vi "read_new_data.vi"(8 "Error In":errorcluster, 9 "connected?":bool, 10 "VISA in":refnum<visa-resource-name>, 11 "Data Cluster In":T1) -> (0 "error out":errorcluster, 2 "VISA out":refnum<visa-resource-name>, 3 "Data Cluster Out":T1)   [LabVIEW 2021]
uses:
  data_cluster_typedef.ctl
panel:
  out "Serial Settings:Number of Bytes at Serial Port":u32
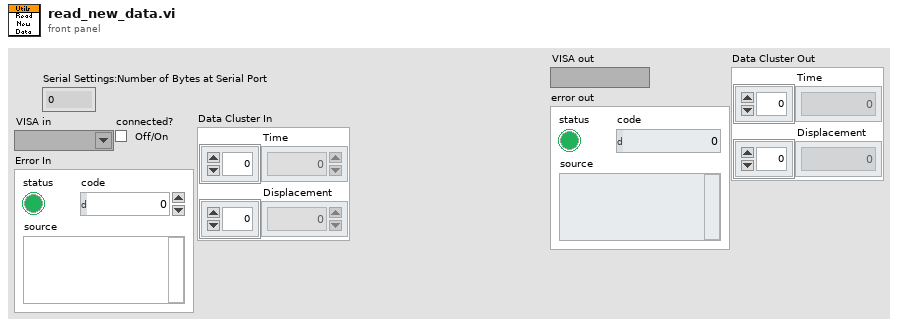
[diagram p1: front panel]
types:
  T1 = typedef "data_cluster_typedef.ctl" = cluster{"Time":dbl[], "Displacement":dbl[]}
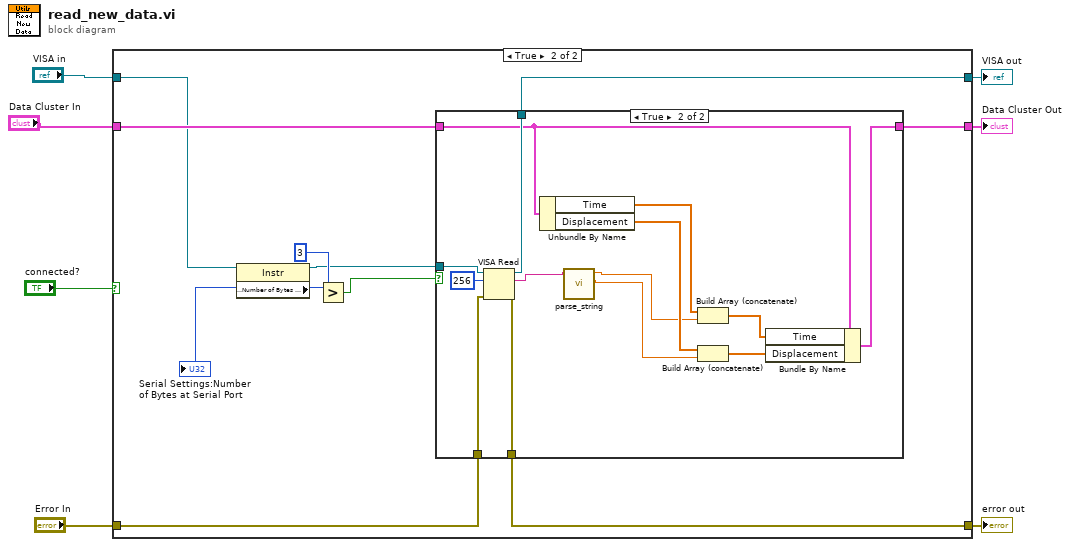
[diagram p0: block diagram]
diagram:
  n1 = case shown="True" "connected?" {
    tunnel: [w10 w20] -> w7
    tunnel: "VISA in" -> [w10 w15]
    tunnel: "Data Cluster In" -> [w9 w18]
    tunnel: [w9 w17] -> w3
    tunnel: "Error In" -> [w8 w19]
    tunnel: [w8 w16] -> w4
    frame False {
      # "Not connected - so just keep passing everything\nthough to keep the graphs, etc populated."
    }
    frame True {
      n2 = property class="Instr"(reference=w15) -> (reference out=w11:refnum<visa-resource-name>, "Serial Settings:Number of Bytes at Serial Port"=w14:u32)  [unwired: 1 in, 1 out]
      "Serial Settings:Number of Bytes at Serial Port" <- w14
      n3 = Greater?(x=w14, y=u32 3) -> (0:w12:bool)
      n4 = case shown="True" w12 {
        tunnel: [w23 w37] -> w20
        tunnel: w19 -> [w22 w36]
        tunnel: w18 -> [w21 w33]
        tunnel: [w21 w32] -> w17
        tunnel: [w22 w31] -> w16
        tunnel: w11 -> [w23 w29]
        frame False {
        }
        frame True {
          n5 = VISA Read(VISA resource name=w29, byte count=u32 256, error in (no error)=w36) -> (VISA resource name out=w37:refnum<visa-resource-name>, read buffer=w26:string, error out=w31:errorcluster)  [unwired: 1 out]
          n6 = Unbundle By Name(w33) -> ("Time"=w35:dbl[], "Displacement"=w34:dbl[])
          n7 = call "parse_string.vi"("Input String"=w26) -> ("Displacement"=w24:dbl, "Time"=w25:dbl)  [unwired: 8 in, 1 out]
          n8 = Build Array (concatenate)(w35, w25) -> (w28:dbl[])
          n9 = Build Array (concatenate)(w34, w24) -> (w27:dbl[])
          n10 = Bundle By Name(cluster=w33, "Time"=w28, "Displacement"=w27) -> (w32:T1)
        }
      }
    }
  }
  "VISA out" <- w7
  "error out" <- w4
  "Data Cluster Out" <- w3
